vi "Set Value.vi"(8 "error in (no error)":errorcluster, 10 "Project Info Value":string, 11 "Item Configuration in":refnum<class "Item Configuration.lvclass">) -> (0 "error out":errorcluster, 3 "Item Configuration out":refnum<class "Item Configuration.lvclass">)   [LabVIEW 2013, in "Item Configuration.lvlib" / "Item Configuration.lvclass"]
uses:
  Item Configuration.lvclass
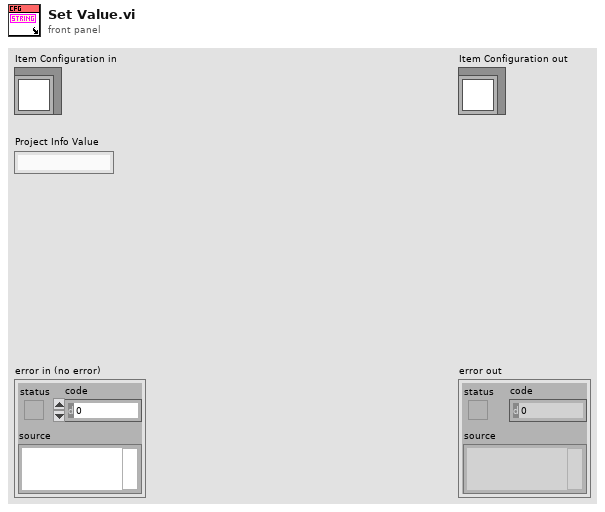
[diagram p1: front panel]
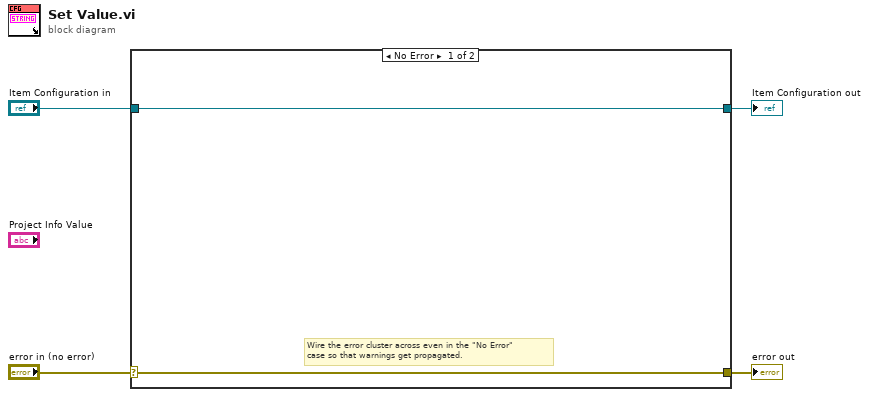
[diagram p0: block diagram]
diagram:
  n1 = case shown="No Error" "error in (no error)" {
    selector: "error in (no error)" -> [w5 w8]
    tunnel: [w5 w8] -> w3
    tunnel: [w6 w7] -> w1
    tunnel: "Item Configuration in" -> [w6 w7]
    frame No Error {
      # "Wire the error cluster across even in the \"No Error\"\ncase so that warnings get propagated."
    }
    frame Error {
    }
  }
  "error out" <- w3
  "Item Configuration out" <- w1
